vi "PADMINI_ZEBRA_PRN_DATA.vi"(6 "QR DATA":string="NB110460ZA210700L27K1234", 7 "DATECODE":string="NB110460ZA210700L27K1234", 8 "error in (no error)":errorcluster, 9 "BBI DESCRIPTION":string="NB110460ZA210700L27K1234", 10 "SERIALNO":string="NB110460ZA210700L27K1234", 11 "BBI PART NO":string="NB110460ZA210700L27K1234") -> (0 "error out":errorcluster, 3 "result PRN":string)   [LabVIEW 2017]
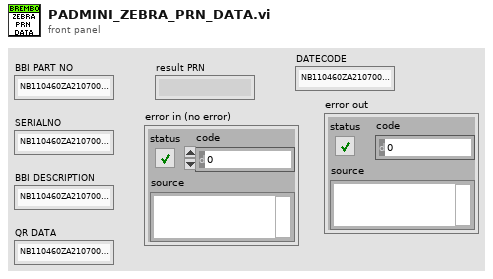
[diagram p1: front panel]
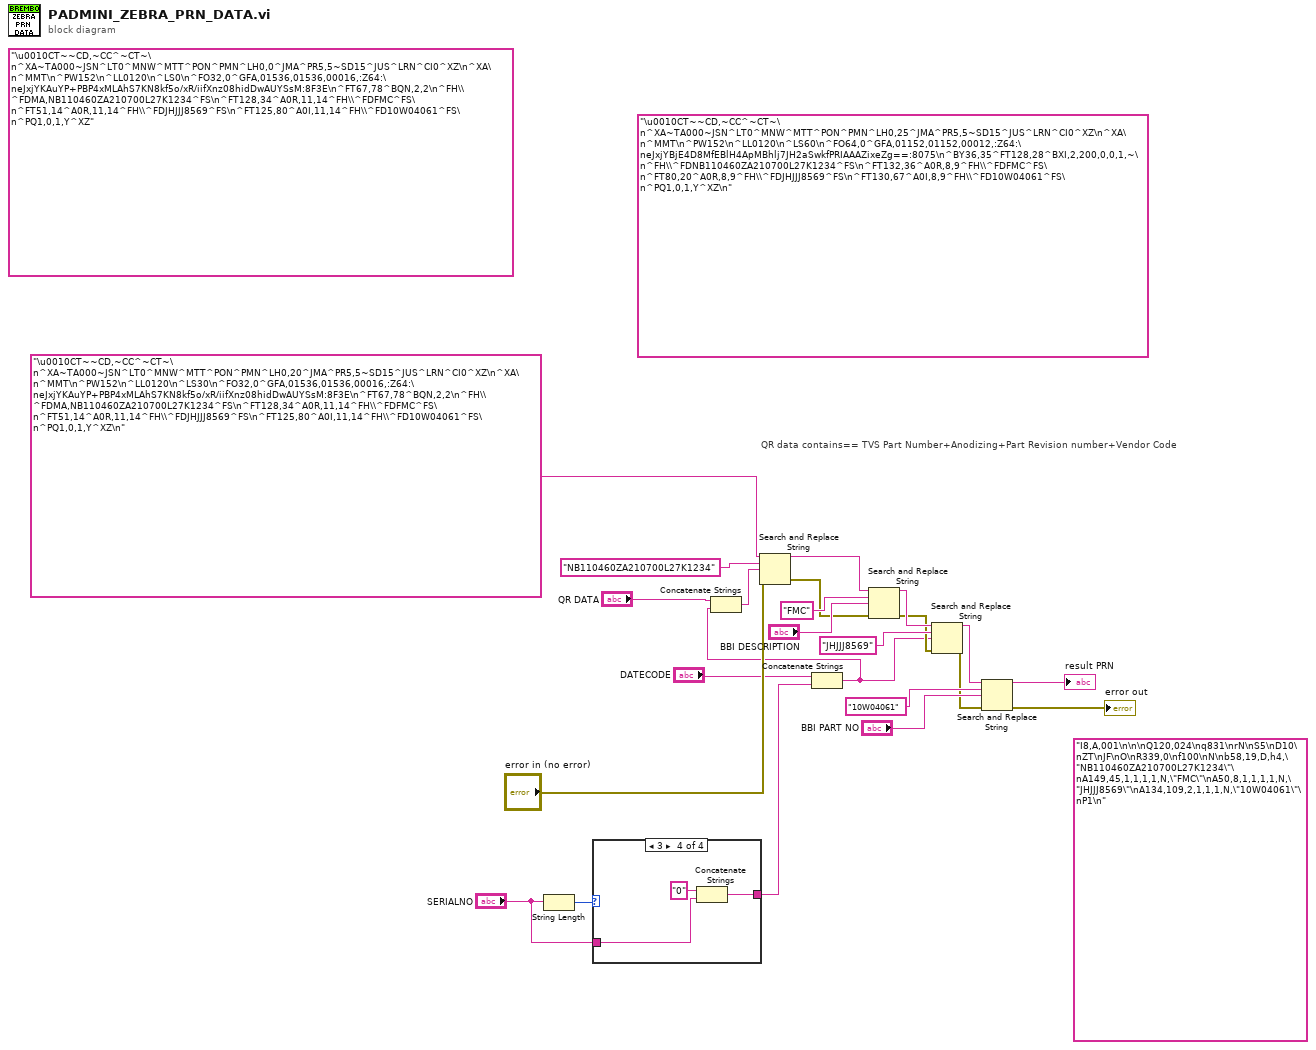
[diagram p0: block diagram]
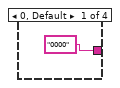
[diagram p2: hidden frame]
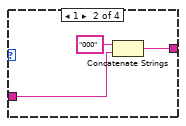
[diagram p3: hidden frame]
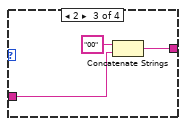
[diagram p4: hidden frame]
diagram:
  (unwired) "\u0010CT~~CD,~CC^~CT~\n^XA~TA000~JSN^LT0^MNW^MTT^PON^PMN^LH0,0^JMA^PR5,5~SD15^JUS^LRN^CI0^XZ\n^XA\n^MMT\n^PW152\n^LL0120\n^LS0\n^FO32,0^GFA,01536,01536,00016,:Z64:\neJxjYKAuYP+PBP4xMLAhS7KN8kf5o/xR/iifXnz08hidDwAUYSsM:8F3E\n^FT67,78^BQN,2,2\n^FH\\^FDMA,NB110460ZA210700L27K1234^FS\n^FT128,34^A0R,11,14^FH\\^FDFMC^FS\n^FT51,14^A0R,11,14^FH\\^FDJHJJJ8569^FS\n^FT125,80^A0I,11,14^FH\\^FD10W04061^FS\n^PQ1,0,1,Y^XZ"
  (unwired) "\u0010CT~~CD,~CC^~CT~\n^XA~TA000~JSN^LT0^MNW^MTT^PON^PMN^LH0,25^JMA^PR5,5~SD15^JUS^LRN^CI0^XZ\n^XA\n^MMT\n^PW152\n^LL0120\n^LS60\n^FO64,0^GFA,01152,01152,00012,:Z64:\neJxjYBjE4D8MfEBlH4ApMBhlj7JH2aSwkfPRIAAAZixeZg==:8075\n^BY36,35^FT128,28^BXI,2,200,0,0,1,~\n^FH\\^FDNB110460ZA210700L27K1234^FS\n^FT132,36^A0R,8,9^FH\\^FDFMC^FS\n^FT80,20^A0R,8,9^FH\\^FDJHJJJ8569^FS\n^FT130,67^A0I,8,9^FH\\^FD10W04061^FS\n^PQ1,0,1,Y^XZ\n"
  (unwired) "I8,A,001\n\n\nQ120,024\nq831\nrN\nS5\nD10\nZT\nJF\nO\nR339,0\nf100\nN\nb58,19,D,h4,\"NB110460ZA210700L27K1234\"\nA149,45,1,1,1,1,N,\"FMC\"\nA50,8,1,1,1,1,N,\"JHJJJ8569\"\nA134,109,2,1,1,1,N,\"10W04061\"\nP1\n"
  # "QR data contains== TVS Part Number+Anodizing+Part Revision number+Vendor Code"
  n1 = String Length(string="SERIALNO") -> (length=w7:i32)
  n2 = case shown="3" w7 {
    tunnel: ["0000" w27 w30 w33] -> w6
    tunnel: "SERIALNO" -> [_ w26 w29 w32]
    frame 0, Default {
    }
    frame 1 {
      n3 = Concatenate Strings("000" ("string"), w26) -> (w27:string)
    }
    frame 2 {
      n4 = Concatenate Strings("00" ("string"), w29) -> (w30:string)
    }
    frame 3 {
      n5 = Concatenate Strings("0" ("string"), w32) -> (w33:string)
    }
  }
  n6 = Concatenate Strings("DATECODE", w6) -> (w4:string)
  n7 = Concatenate Strings("QR DATA", w4) -> (w2:string)
  n8 = Search and Replace String(input string="\u0010CT~~CD,~CC^~CT~\n^XA~TA000~JSN^LT0^MNW^MTT^PON^PMN^LH0,20^JMA^PR5,5~SD15^JUS^LRN^CI0^XZ\n^XA\n^MMT\n^PW152\n^LL0120\n^LS30\n^FO32,0^GFA,01536,01536,00016,:Z64:\neJxjYKAuYP+PBP4xMLAhS7KN8kf5o/xR/iifXnz08hidDwAUYSsM:8F3E\n^FT67,78^BQN,2,2\n^FH\\^FDMA,NB110460ZA210700L27K1234^FS\n^FT128,34^A0R,11,14^FH\\^FDFMC^FS\n^FT51,14^A0R,11,14^FH\\^FDJHJJJ8569^FS\n^FT125,80^A0I,11,14^FH\\^FD10W04061^FS\n^PQ1,0,1,Y^XZ\n", search string="NB110460ZA210700L27K1234" ("regular expression"), replace string=w2, error in="error in (no error)") -> (result string=w15:string, error out=w12:errorcluster)  [unwired: 4 in, 2 out]
  n9 = Search and Replace String(input string=w15, search string="FMC" ("regular expression"), replace string="BBI DESCRIPTION", error in=w12) -> (result string=w18:string, error out=w11:errorcluster)  [unwired: 4 in, 2 out]
  n10 = Search and Replace String(input string=w18, search string="JHJJJ8569" ("regular expression"), replace string=w4, error in=w11) -> (result string=w20:string, error out=w10:errorcluster)  [unwired: 4 in, 2 out]
  n11 = Search and Replace String(input string=w20, search string="10W04061" ("regular expression"), replace string="BBI PART NO", error in=w10) -> (result string=→"result PRN":string, error out=→"error out":errorcluster)  [unwired: 4 in, 2 out]
